vi "Example 1.vi"() -> ()   [LabVIEW 2026, in "VFD Library.lvlib"]
uses:
  VFD Library.lvlib
  Public/Action/Direction Selection.ctl
panel:
  in  "RESET":bool
  out "Faults":string[](array[string])
  out "Fault":bool
  out "Motor feedback\nspeed":dbl format="%#_13g"
  out "error out":errorcluster
  in  "Stop":bool
  out "Current":dbl format="%#_13g"
  out "Voltage":dbl format="%#_13g"
  in  "Direction":T1=2 items=["Reverse"=0, "Forward"=2]
  in  "Set Deceleration time":u16=5
  in  "Set Acceleration time":u16=5
  in  "Enable":bool
  in  "Set RPM":u16
  in  "IP Address":string="172.20.0.115"
  # "VFD MANUAL CONTROL"
  # "Configuration"
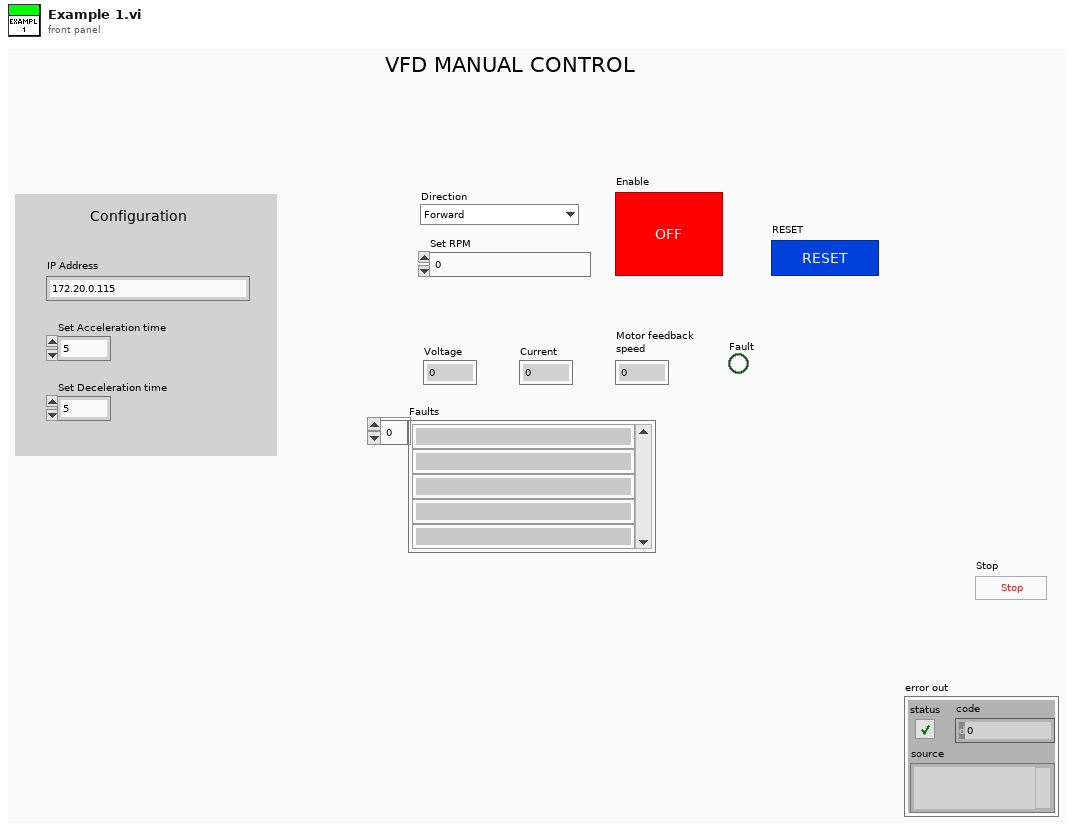
[diagram p1: front panel]
types:
  T1 = typedef "VFD Library.lvlib/Direction Selection.ctl" = u16
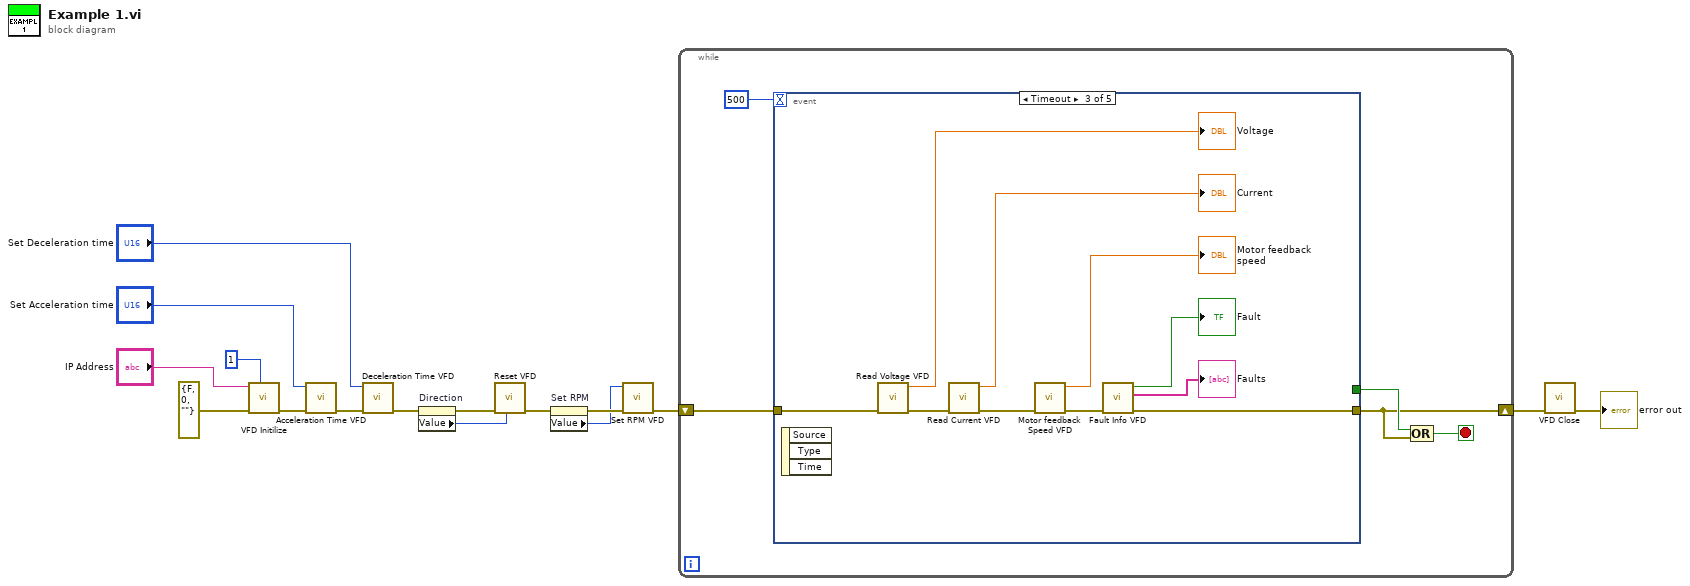
[diagram p0: block diagram]
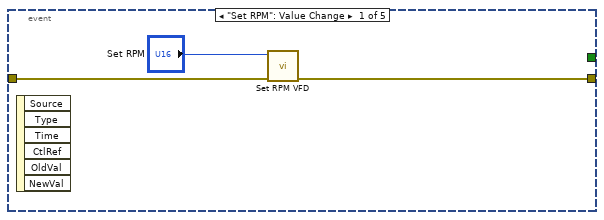
[diagram p2: hidden frame]
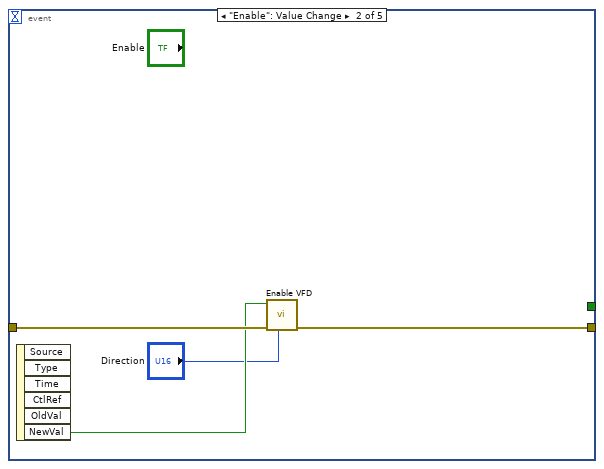
[diagram p3: hidden frame]
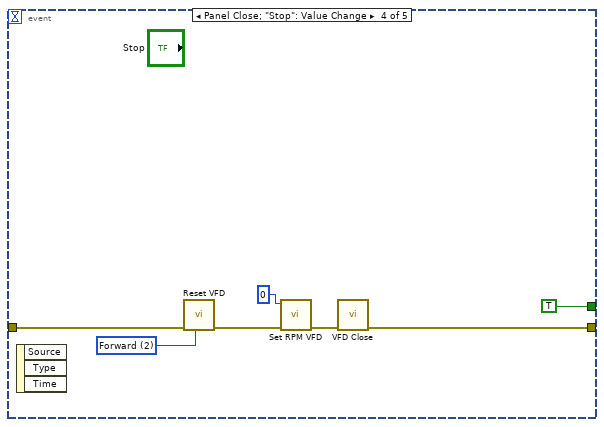
[diagram p4: hidden frame]
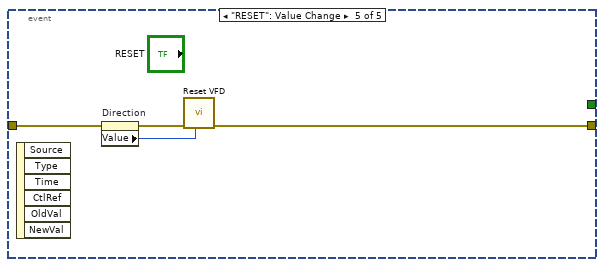
[diagram p5: hidden frame]
diagram:
  n1 = call "VFD Initilize.vi"("Slave ID (255)"=u8 1, "error In"=errorcluster {"status"=FALSE, "code"=0, "source"=""}, "IP Address"="IP Address") -> ("error out"=w14:errorcluster)  [unwired: 8 in]
  n2 = call "Acceleration Time VFD.vi"("error In"=w14, "Set Acceleration time"="Set Acceleration time") -> ("error out"=w13:errorcluster)  [unwired: 9 in]
  n3 = call "Deceleration Time VFD.vi"("error In"=w13, "Set Deceleration time"="Set Deceleration time") -> ("error out"=w6:errorcluster)  [unwired: 9 in]
  n4 = property on="Direction" class="Ring (strict)"(error in=w6) -> (error out=w5:errorcluster, "Value"=w4:T1)  [unwired: 1 in, 1 out]
  n5 = call "Reset VFD.vi"("Direction"=w4, "error In"=w5) -> ("error out"=w3:errorcluster)  [unwired: 9 in]
  n6 = property on="Set RPM" class="DigNum (strict)"(error in=w3) -> (error out=w2:errorcluster, "Value"=w1:u16)  [unwired: 1 in, 1 out]
  n7 = call "Set RPM VFD.vi"("error In"=w2, "Set RPM"=w1) -> ("error out"=w11:errorcluster)  [unwired: 9 in]
  n8 = while {
    shift-right: [w17] -> w9
    shift-left: w11 -> [w21]
    stop <- w18 stop-if-true
    n9 = event shown="[2] Timeout" {
      selector: _ -> [_ _ _ _ _]
      dyn-events: _ -> [_ _ _ _ _]
      timeout: 500 -> [_ _ _ _ _]
      tunnel: w21 -> [w24 w28 w38 w45 w48]
      tunnel: [w23 w27 w31 w44 w49] -> w17
      tunnel: [_ _ _ TRUE _] -> w19
      event "Set RPM": Value Change {
        n10 = event-data() -> ()  [unwired: 1 in, 6 out]
        n11 = call "Set RPM VFD.vi"("error In"=w24, "Set RPM"="Set RPM") -> ("error out"=w23:errorcluster)  [unwired: 9 in]
      }
      event "Enable": Value Change {
        n12 = event-data() -> ("NewVal"=w26:bool)  [unwired: 1 in, 5 out]
        n13 = call "Enable VFD.vi"("Direction"="Direction", "error In"=w28, "Enable"=w26) -> ("error out"=w27:errorcluster)  [unwired: 8 in]
      }
      event Timeout {
        n14 = event-data() -> ()  [unwired: 1 in, 3 out]
        n15 = call "Read Voltage VFD.vi"("error In"=w38) -> ("error out"=w37:errorcluster, "Voltage"=→"Voltage":dbl)  [unwired: 9 in]
        n16 = call "Read Current VFD.vi"("error In"=w37) -> ("error out"=w34:errorcluster, "Current"=→"Current":dbl)  [unwired: 9 in]
        n17 = call "Motor feedback Speed VFD.vi"("error In"=w34) -> ("error out"=w32:errorcluster, "Motor feedback\nspeed"=→"Motor feedback\nspeed":dbl)  [unwired: 9 in]
        n18 = call "Fault Info VFD.vi"("error In"=w32) -> ("error out"=w31:errorcluster, "Faults"=→"Faults":string[], "Fault"=→"Fault":bool)  [unwired: 8 in]
      }
      event Panel Close; "Stop": Value Change {
        w43 = T1 2 items=["Reverse"=0, "Forward"=2] ("Direction")
        n19 = event-data() -> ()  [unwired: 1 in, 3 out]
        n20 = call "Reset VFD.vi"("Direction"=w43, "error In"=w45) -> ("error out"=w41:errorcluster)  [unwired: 9 in]
        n21 = call "Set RPM VFD.vi"("error In"=w41, "Set RPM"=u16 0) -> ("error out"=w40:errorcluster)  [unwired: 9 in]
        n22 = call "VFD Close.vi"("error In"=w40) -> ("error out"=w44:errorcluster)  [unwired: 10 in]
      }
      event "RESET": Value Change {
        n23 = event-data() -> ()  [unwired: 1 in, 6 out]
        n24 = property on="Direction" class="Ring (strict)"(error in=w48) -> (error out=w47:errorcluster, "Value"=w46:T1)  [unwired: 1 in, 1 out]
        n25 = call "Reset VFD.vi"("Direction"=w46, "error In"=w47) -> ("error out"=w49:errorcluster)  [unwired: 9 in]
      }
    }
    n26 = Compound Arithmetic op=OR(w19, w17) -> (w18:bool)
  }
  n27 = call "VFD Close.vi"("error In"=w9) -> ("error out"=→"error out":errorcluster)  [unwired: 10 in]
